vi "Blink User1 LED.vi"() -> ()   [LabVIEW 2025]
uses:
  <vilib>/NI_Real-Time Target Support.lvlib
panel:
  out "LED State":bool
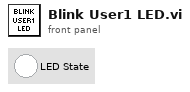
[diagram p1: front panel]
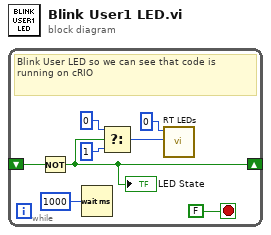
[diagram p0: block diagram]
diagram:
  n1 = while {
    shift-right: [w3] -> _
    shift-left: _ -> [w2]
    stop <- FALSE stop-if-true
    # "Blink User LED so we can see that code is running on cRIO"
    n2 = Not(x=w2) -> (.not. x?=w3:bool)
    "LED State" <- w3
    n3 = Wait (ms)(milliseconds to wait=u32 1000) -> ()  [unwired: 1 out]
    n4 = Select(t=0 ("State"), s=w3, f=1 ("State")) -> (s? t:f=w4:i32)
    n5 = call <vilib>:"RT LEDs.vi"("State"=w4, "LED Num"=0) -> ()  [unwired: 4 in, 2 out]
  }
